vi "All Child Values.vi"(11 "Game in":refnum<class "Game.lvclass">) -> (2 "All Values":refnum<class "Type.lvclass">[](array[class]))   [LabVIEW 2020, in "Conditum-Example.lvlib" / "Game.lvclass"]
uses:
  Game.lvclass
  Conditum/Columns/Type/Type.lvclass
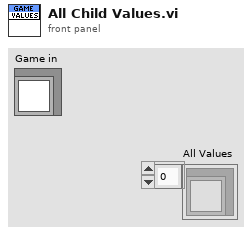
[diagram p1: front panel]
types:
  T1 = typedef "Conditum-Example.lvlib/Game.lvclass/Columns.ctl" = cluster{"Owner":refnum<class "Entity C.lvclass">, "Players":refnum<class "Entity Collection.lvclass">, "Name":refnum<class "String.lvclass">, "Started":refnum<class "Timestamp.lvclass">, "Completed":refnum<class "Boolean.lvclass">}
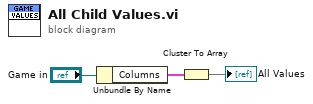
[diagram p0: block diagram]
diagram:
  n1 = Unbundle By Name("Game in") -> ("Columns"=w2:T1)
  n2 = Cluster To Array(cluster=w2) -> (array=→"All Values":refnum<class "Type.lvclass">[])
